vi "Read CSV File.vi"(8 "error in":errorcluster) -> (0 "error out":errorcluster, 3 "Zone Setup Array":cluster{"Zone Selector":string, "Timing":dbl}[](array[cluster]))   [LabVIEW 2020]
doc: "This VI reads the CSV file provided and updates the Zone Setup Array."
uses:
  <vilib>/Utility/file.llb/Read Delimited Spreadsheet (string).vi
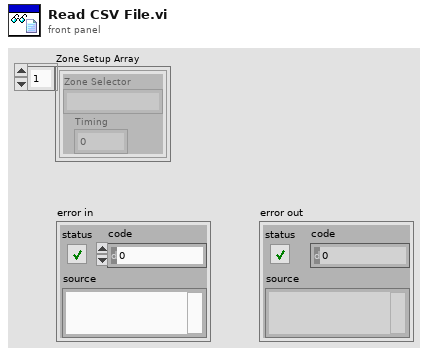
[diagram p1: front panel]
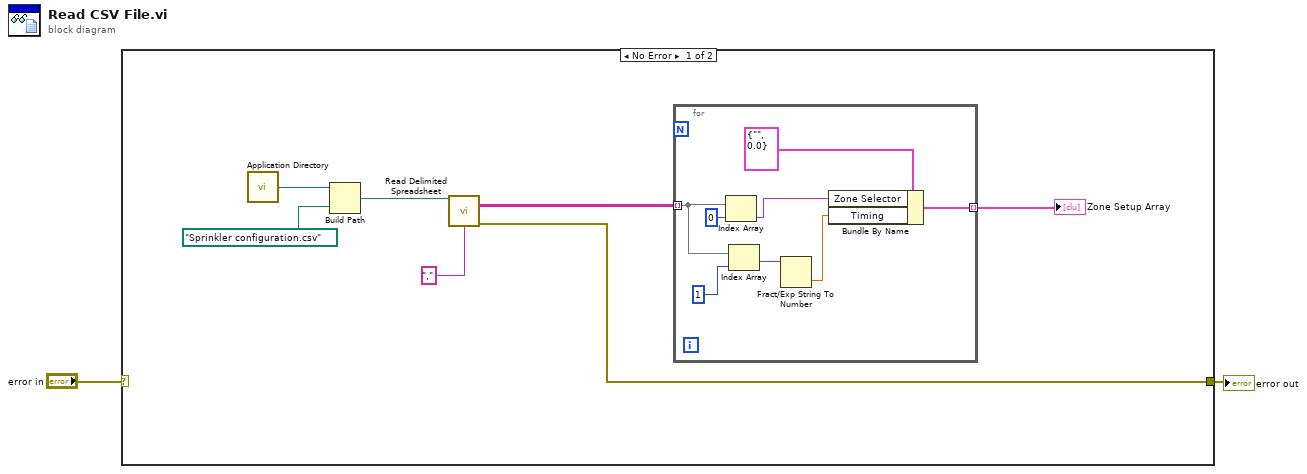
[diagram p0: block diagram]
diagram:
  n1 = case shown="No Error" "error in" {
    selector: "error in" -> [_ w18]
    tunnel: [w3 w18] -> w2
    frame No Error {
      n2 = call <vilib>:"Application Directory.vi"() -> ("Application Directory"=w4:path)
      n3 = Build Path(base path=w4, name or relative path=path "Sprinkler configuration.csv") -> (appended path=w6:path)
      n4 = call-poly <vilib>:"Read Delimited Spreadsheet.vi"("file path (dialog if empty)"=w6, "delimiter (\\t)"="," ("delimiter (\\t)")) -> ("all rows"=w8:string[][], "error out"=w3:errorcluster)  [unwired: 8 in, 4 out]
      n5 = for {
        tunnel: w8 -> [w12] mode=indexing
        tunnel: [w17] -> w9 mode=indexing
        n6 = Index Array(array=w12, index=0) -> (element=w15:string)
        n7 = Index Array(array=w12, index=1) -> (element=w13:string)
        n8 = Fract/Exp String To Number(string=w13) -> (number=w11:dbl)  [unwired: 3 in, 1 out]
        n9 = Bundle By Name(cluster=cluster{"Zone Selector":string, "Timing":dbl} {"Zone Selector"="", "Timing"=0.0} ("Zone Selector"), "Zone Selector"=w15, "Timing"=w11) -> (w17:cluster{"Zone Selector":string, "Timing":dbl})
      }
      "Zone Setup Array" <- w9
    }
    frame Error {
    }
  }
  "error out" <- w2
